vi "Read Section Fuel.vi"(11 "section in":string="S1") -> (3 "Data Cluster":T1)   [LabVIEW 2017, in "Konfiguracja.lvlib"]
uses:
  Konfiguracja.lvlib
  <vilib>/Utility/config.llb/NI_LVConfig.lvlib
panel:
  in  "P_Rx":T2
  in  "P_Sx":T3
  in  "Px":T4
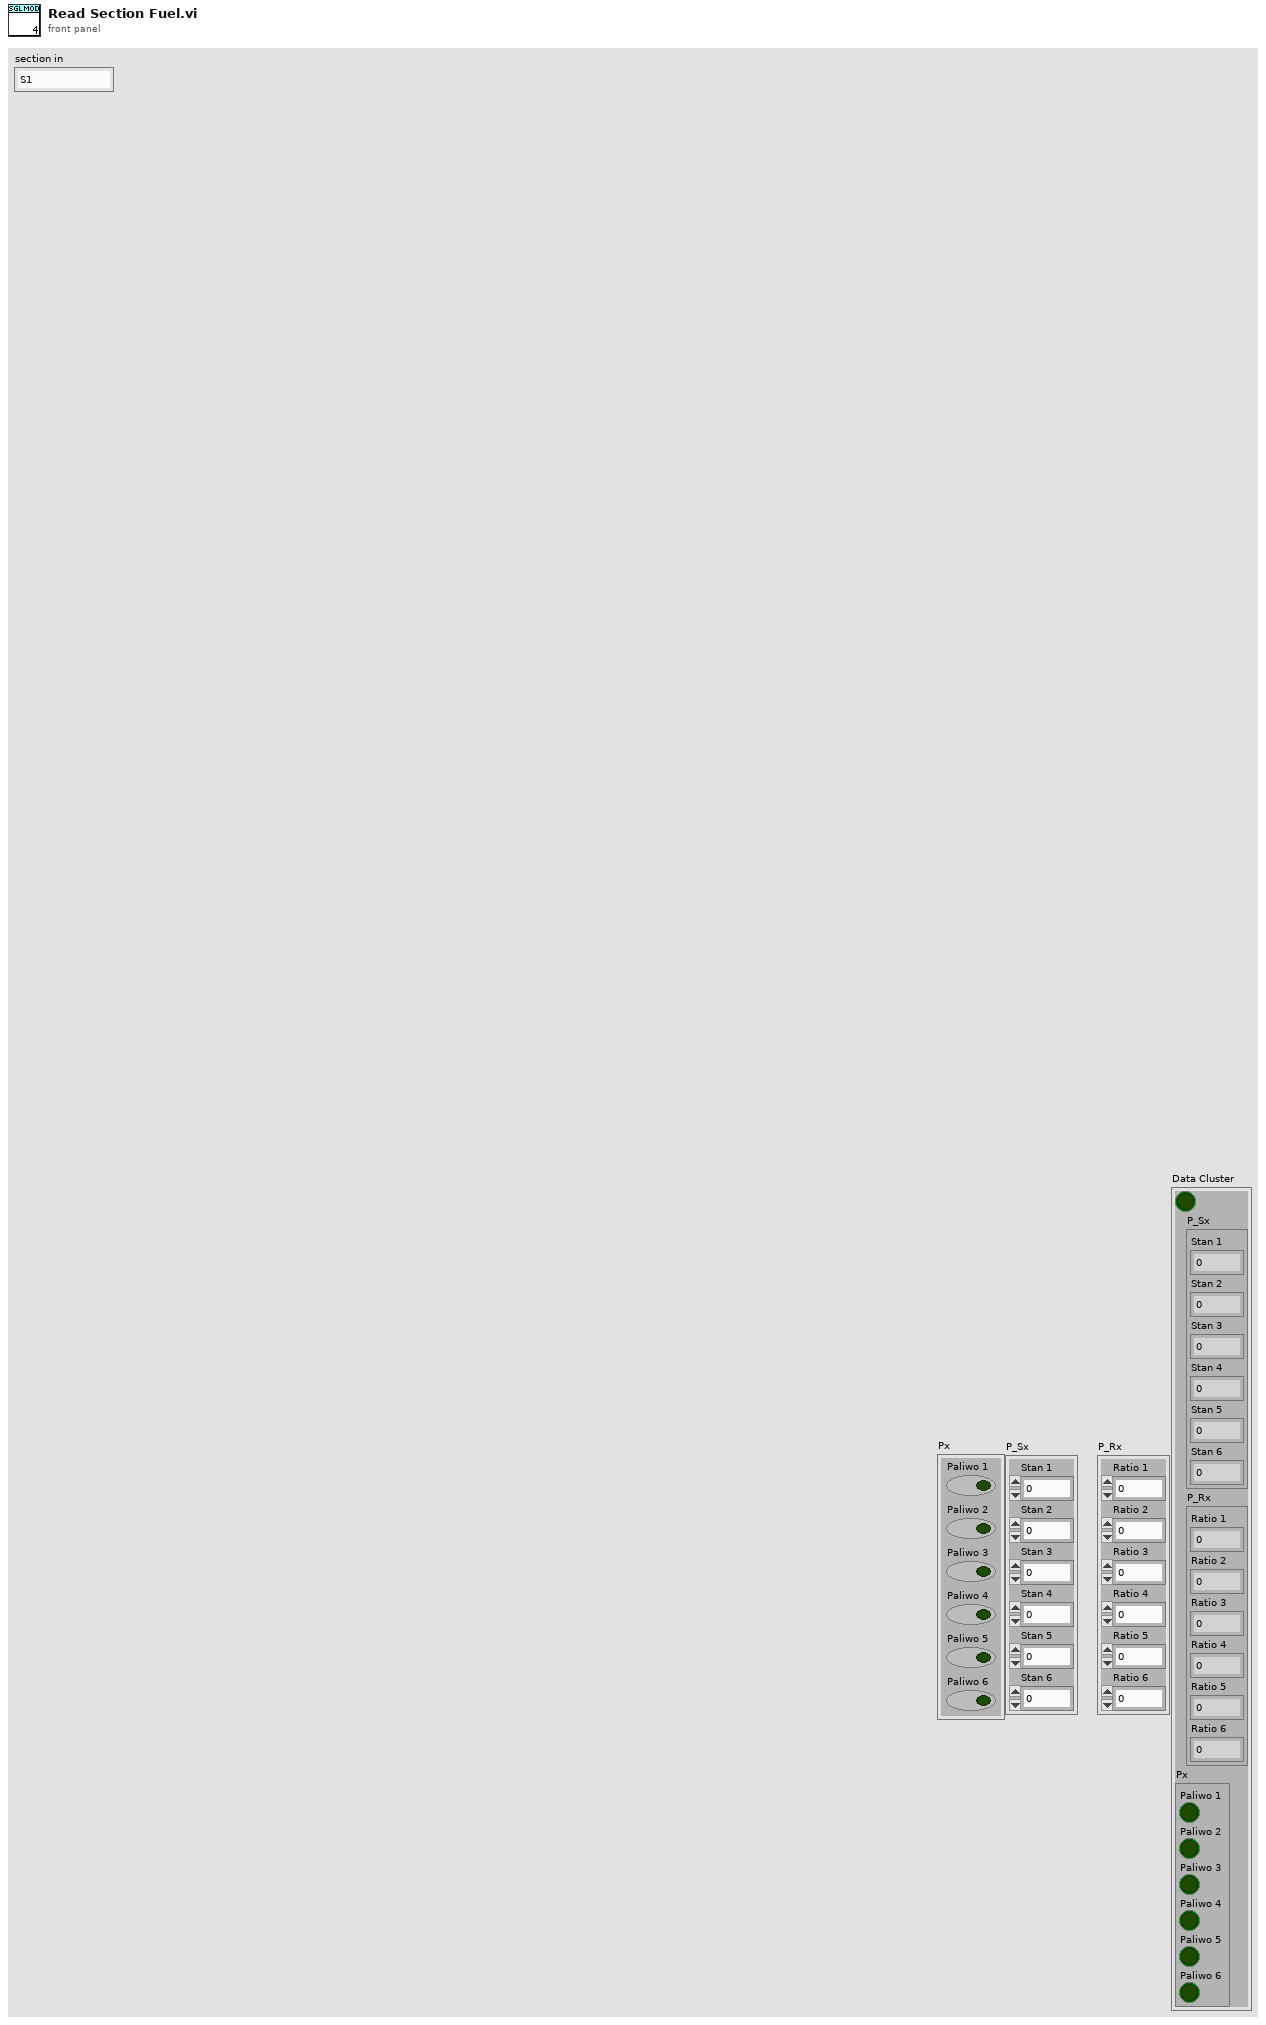
[diagram p1: front panel]
types:
  T1 = cluster{bool, "P_Sx":cluster{"Stan 1":dbl, "Stan 2":dbl, "Stan 3":dbl, "Stan 4":dbl, "Stan 5":dbl, "Stan 6":dbl}, "P_Rx":cluster{"Ratio 1":dbl, "Ratio 2":dbl, "Ratio 3":dbl, "Ratio 4":dbl, "Ratio 5":dbl, "Ratio 6":dbl}, "Px":cluster{"Paliwo 1":bool, "Paliwo 2":bool, "Paliwo 3":bool, "Paliwo 4":bool, "Paliwo 5":bool, "Paliwo 6":bool}}
  T2 = cluster{"Ratio 1":dbl, "Ratio 2":dbl, "Ratio 3":dbl, "Ratio 4":dbl, "Ratio 5":dbl, "Ratio 6":dbl}
  T3 = cluster{"Stan 1":dbl, "Stan 2":dbl, "Stan 3":dbl, "Stan 4":dbl, "Stan 5":dbl, "Stan 6":dbl}
  T4 = cluster{"Paliwo 1":bool, "Paliwo 2":bool, "Paliwo 3":bool, "Paliwo 4":bool, "Paliwo 5":bool, "Paliwo 6":bool}
  T5 = typedef "NI_LVConfig.lvlib/Config Data RefNum.ctl" = refnum<k1>
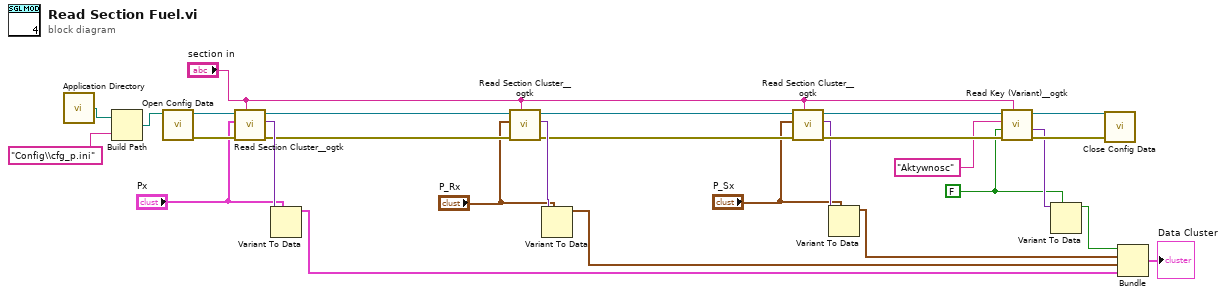
[diagram p0: block diagram]
diagram:
  w21 = FALSE
  n1 = call <vilib>:"Application Directory.vi"() -> ("Application Directory"=w15:path)
  n2 = Build Path(base path=w15, name or relative path="Config\\cfg_p.ini") -> (appended path=w13:path)
  n3 = call <vilib>:"Open Config Data.vi"("configuration file path"=w13) -> ("error out"=w7:errorcluster, "refnum"=w19:T5)  [unwired: 8 in, 1 out]
  n4 = call <userlib>:"Read Section Cluster__ogtk.vi"("section (optional)"="section in", "error in (no error)"=w7, "Section Formatted Cluster Type"="Px", "refnum"=w19) -> ("error out"=w6:errorcluster, "Section Formatted Cluster"=w10:variant, "dup refnum"=w12:T5)  [unwired: 3 in, 2 out]
  n5 = Variant To Data(type="Px", Variant=w10) -> (data=w16:T4)  [unwired: 1 in, 1 out]
  n6 = call <userlib>:"Read Section Cluster__ogtk.vi"("section (optional)"="section in", "error in (no error)"=w6, "Section Formatted Cluster Type"="P_Rx", "refnum"=w12) -> ("error out"=w5:errorcluster, "Section Formatted Cluster"=w9:variant, "dup refnum"=w11:T5)  [unwired: 3 in, 2 out]
  n7 = Variant To Data(type="P_Rx", Variant=w9) -> (data=w17:T2)  [unwired: 1 in, 1 out]
  n8 = call <userlib>:"Read Section Cluster__ogtk.vi"("section (optional)"="section in", "error in (no error)"=w5, "Section Formatted Cluster Type"="P_Sx", "refnum"=w11) -> ("error out"=w25:errorcluster, "Section Formatted Cluster"=w8:variant, "dup refnum"=w24:T5)  [unwired: 3 in, 2 out]
  n9 = Variant To Data(type="P_Sx", Variant=w8) -> (data=w18:T3)  [unwired: 1 in, 1 out]
  n10 = call <userlib>:"Read Key (Variant)__ogtk.vi"("section"="section in", "error in (no error)"=w25, "type"=w21, "key (optional)"="Aktywnosc", "refnum"=w24) -> ("error out"=w28:errorcluster, "key-value"=w22:variant, "refnum out"=w27:T5)  [unwired: 3 in, 1 out]
  n11 = Variant To Data(type=w21, Variant=w22) -> (data=w26:bool)  [unwired: 1 in, 1 out]
  n12 = call <vilib>:"Close Config Data.vi"("error in (no error)"=w28, "refnum"=w27) -> ()  [unwired: 8 in, 2 out]
  n13 = Bundle(w26, "P_Sx"=w18, "P_Rx"=w17, "Px"=w16) -> (→"Data Cluster":T1)  [unwired: 1 in]
